vi "Get_value_from_OPC.vi"(8 "Address to read":string, 9 "OPC UA client refnum in":T1) -> (1 "Timestamp":timestamp, 2 "Data out":variant, 3 "OPC UA client refnum out":T1)   [LabVIEW 2021]
uses:
  <vilib>/OPCUA/controls/OPC UA Client Refnum.ctl
  <vilib>/OPCUA/client/Multiple Read Variant.vi
  <vilib>/OPCUA/NI OPC UA Client.lvlib
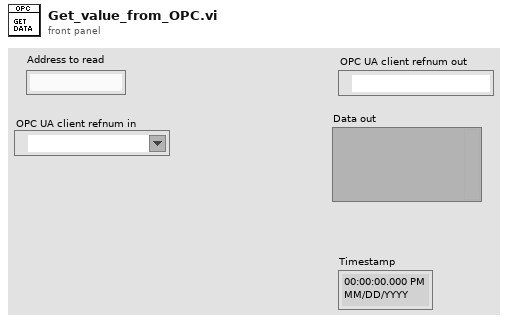
[diagram p1: front panel]
types:
  T1 = typedef "OPC UA Client Refnum.ctl" = refnum<k21>
  T2 = typedef "Read Variant Result.ctl" = cluster{"node ID":T3, "value ":variant, "timestamp":timestamp, "status":T4}
  T3 = typedef "NodeId.ctl" = string
  T4 = typedef "OPC UA StatusCode.ctl" = u32
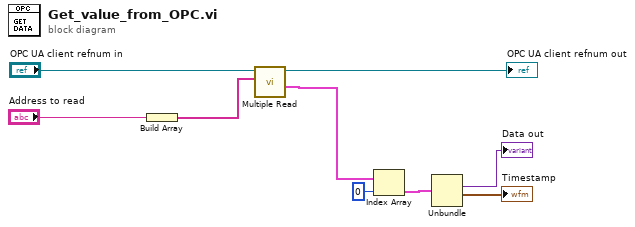
[diagram p0: block diagram]
diagram:
  n1 = Build Array("Address to read") -> (w3:string[])
  n2 = call-poly <vilib>:"Multiple Read.vi"("node IDs"=w3, "OPC UA client refnum in"="OPC UA client refnum in") -> ("results"=w2:T2[], "OPC UA client refnum out"=→"OPC UA client refnum out":T1)  [unwired: 6 in, 2 out]
  n3 = Index Array(array=w2, index=0) -> (element=w8:T2)
  n4 = Unbundle(w8) -> ("value"=→"Data out":variant, "timestamp"=→"Timestamp":timestamp)  [unwired: 2 out]
